vi "Perform File Operations.vi"(0 "VISA resource name":refnum<visa-resource-name>, 1 "File Operation(0:Copy)":i32(ring) items=["Copy", "Move", "Delete"], 5 "File Type (0:Hard Copy)":i32(ring) items=["Hard Copy", "Parameter", "System Info", "Trace"], 7 "Application (0:Spectrum Analyzer)":i32(ring) items=["Spectrum Analyzer", "Phase Noise"], 9 "Filename (TEST)":string="TEST", 11 "error in (no error)":errorcluster, 12 "Driver Letter (D)":string="D") -> (4 "VISA resource name out":refnum<visa-resource-name>, 15 "error out":errorcluster)   [LabVIEW 2020, in "Anritsu Signal Analyzer Series.lvlib"]
doc: "Copies , Moves, or Deletes a screen hardcopy, parameter file copied in the internal hard disk , system information file, or a trace file copied in the internal hard disk to the specified device."
uses:
  Anritsu Signal Analyzer Series.lvlib
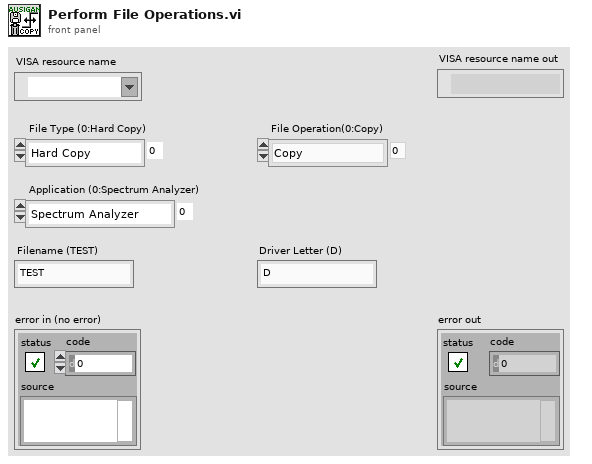
[diagram p1: front panel]
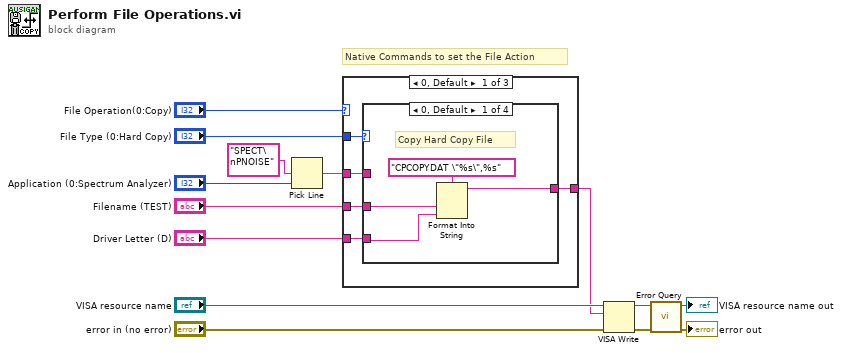
[diagram p0: block diagram]
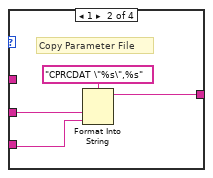
[diagram p2: hidden frame]
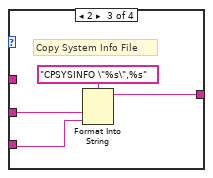
[diagram p3: hidden frame]
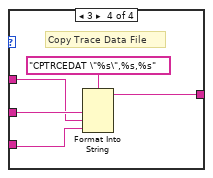
[diagram p4: hidden frame]
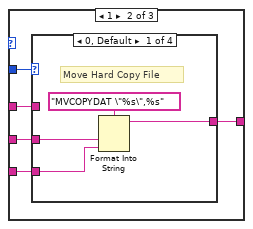
[diagram p5: hidden frame]
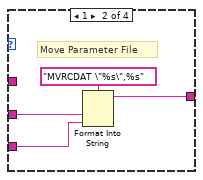
[diagram p6: hidden frame]
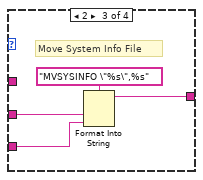
[diagram p7: hidden frame]
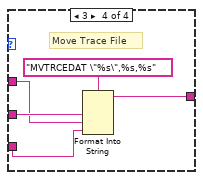
[diagram p8: hidden frame]
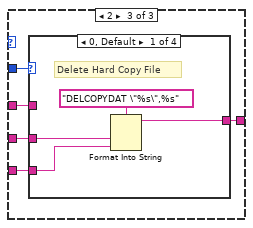
[diagram p9: hidden frame]
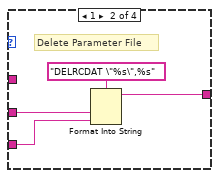
[diagram p10: hidden frame]
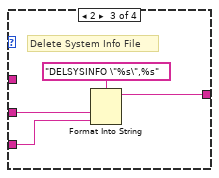
[diagram p11: hidden frame]
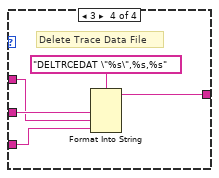
[diagram p12: hidden frame]
diagram:
  # "Native Commands to set the File Action"
  n1 = Pick Line(multi-line string="SPECT\nPNOISE", line index="Application (0:Spectrum Analyzer)") -> (output string=w2:string)  [unwired: 1 in]
  n2 = case shown="0, Default" "File Operation(0:Copy)" {
    tunnel: "File Type (0:Hard Copy)" -> [w19 w41 w63]
    tunnel: "Driver Letter (D)" -> [w18 w39 w61]
    tunnel: "Filename (TEST)" -> [w17 w40 w62]
    tunnel: [w16 w38 w60] -> w5
    tunnel: w2 -> [w15 w37 w59]
    frame 0, Default {
      n3 = case shown="0, Default" w19 {
        tunnel: w17 -> [w23 w27 w31 w36]
        tunnel: w18 -> [w22 w26 w30 w33]
        tunnel: w15 -> [_ _ _ w32]
        tunnel: [w20 w24 w28 w34] -> w16
        frame 0, Default {
          # "Copy Hard Copy File"
          n4 = Format Into String(format string="CPCOPYDAT \"%s\",%s" ("_Command"), w23, w22) -> (resulting string=w20:string)  [unwired: 2 in, 1 out]
        }
        frame 1 {
          # "Copy Parameter File"
          n5 = Format Into String(format string="CPRCDAT \"%s\",%s" ("_Command"), w27, w26) -> (resulting string=w24:string)  [unwired: 2 in, 1 out]
        }
        frame 2 {
          # "Copy System Info File"
          n6 = Format Into String(format string="CPSYSINFO \"%s\",%s" ("_Command"), w31, w30) -> (resulting string=w28:string)  [unwired: 2 in, 1 out]
        }
        frame 3 {
          # "Copy Trace Data File"
          n7 = Format Into String(format string="CPTRCEDAT \"%s\",%s,%s" ("_Command"), w36, w32, w33) -> (resulting string=w34:string)  [unwired: 2 in, 1 out]
        }
      }
    }
    frame 1 {
      n8 = case shown="0, Default" w41 {
        tunnel: w40 -> [w45 w49 w53 w58]
        tunnel: w39 -> [w44 w48 w52 w55]
        tunnel: [w42 w46 w50 w56] -> w38
        tunnel: w37 -> [_ _ _ w54]
        frame 0, Default {
          # "Move Hard Copy File"
          n9 = Format Into String(format string="MVCOPYDAT \"%s\",%s" ("_Command"), w45, w44) -> (resulting string=w42:string)  [unwired: 2 in, 1 out]
        }
        frame 1 {
          # "Move Parameter File"
          n10 = Format Into String(format string="MVRCDAT \"%s\",%s" ("_Command"), w49, w48) -> (resulting string=w46:string)  [unwired: 2 in, 1 out]
        }
        frame 2 {
          # "Move System Info File"
          n11 = Format Into String(format string="MVSYSINFO \"%s\",%s" ("_Command"), w53, w52) -> (resulting string=w50:string)  [unwired: 2 in, 1 out]
        }
        frame 3 {
          # "Move Trace File"
          n12 = Format Into String(format string="MVTRCEDAT \"%s\",%s,%s" ("_Command"), w58, w54, w55) -> (resulting string=w56:string)  [unwired: 2 in, 1 out]
        }
      }
    }
    frame 2 {
      n13 = case shown="0, Default" w63 {
        tunnel: w62 -> [w67 w71 w75 w80]
        tunnel: w61 -> [w66 w70 w74 w77]
        tunnel: w59 -> [_ _ _ w76]
        tunnel: [w64 w68 w72 w78] -> w60
        frame 0, Default {
          # "Delete Hard Copy File"
          n14 = Format Into String(format string="DELCOPYDAT \"%s\",%s" ("_Command"), w67, w66) -> (resulting string=w64:string)  [unwired: 2 in, 1 out]
        }
        frame 1 {
          # "Delete Parameter File"
          n15 = Format Into String(format string="DELRCDAT \"%s\",%s" ("_Command"), w71, w70) -> (resulting string=w68:string)  [unwired: 2 in, 1 out]
        }
        frame 2 {
          # "Delete System Info File"
          n16 = Format Into String(format string="DELSYSINFO \"%s\",%s" ("_Command"), w75, w74) -> (resulting string=w72:string)  [unwired: 2 in, 1 out]
        }
        frame 3 {
          # "Delete Trace Data File"
          n17 = Format Into String(format string="DELTRCEDAT \"%s\",%s,%s" ("_Command"), w80, w76, w77) -> (resulting string=w78:string)  [unwired: 2 in, 1 out]
        }
      }
    }
  }
  n18 = VISA Write(VISA resource name="VISA resource name", write buffer=w5, error in (no error)="error in (no error)") -> (VISA resource name out=w6:refnum<visa-resource-name>, error out=w7:errorcluster)  [unwired: 1 out]
  n19 = call "Error Query.vi"("error in (no error)"=w7, "VISA resource name"=w6) -> ("error out"=→"error out":errorcluster, "VISA resource name out"=→"VISA resource name out":refnum<visa-resource-name>)  [unwired: 6 in, 2 out]
